vi "Keep time between injections.vi"(6 "Boolean in":bool, 9 "Current Element":string, 10 "Time Target for last measurement in":dbl, 11 "Item Names":string[](array[string])) -> (2 "Boolean out":bool, 3 "Elapsed Time (s)":dbl)   [LabVIEW 2014]
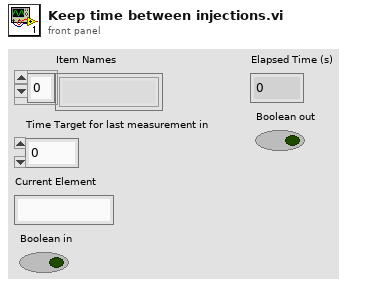
[diagram p1: front panel]
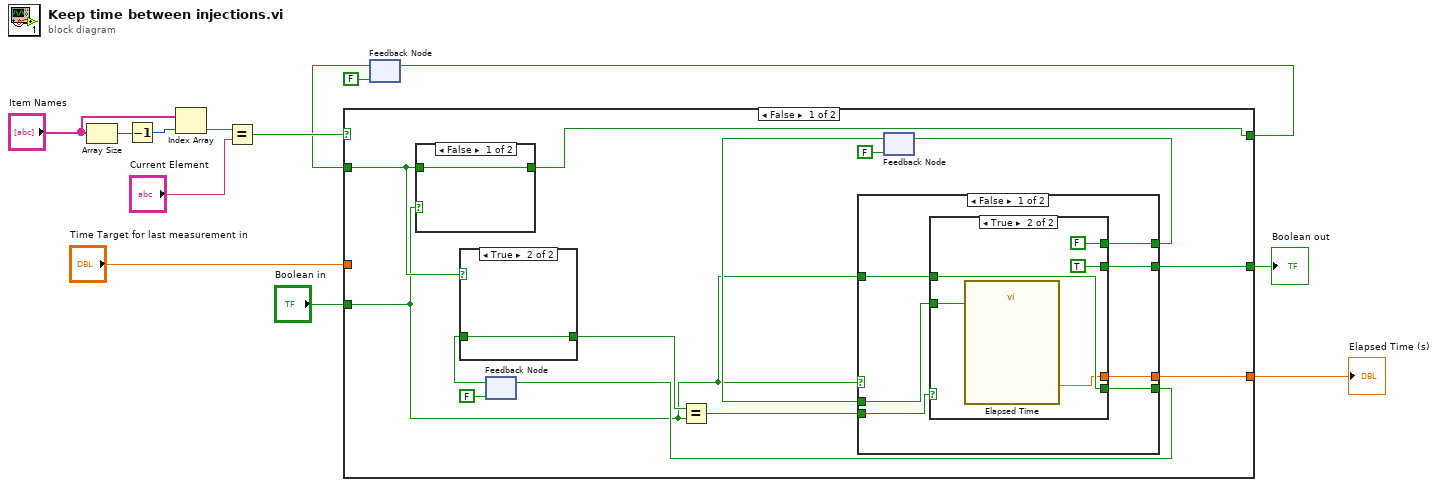
[diagram p0: block diagram]
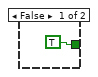
[diagram p2: hidden frame]
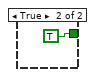
[diagram p3: hidden frame]
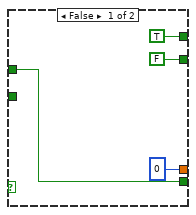
[diagram p4: hidden frame]
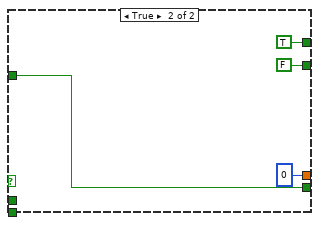
[diagram p5: hidden frame]
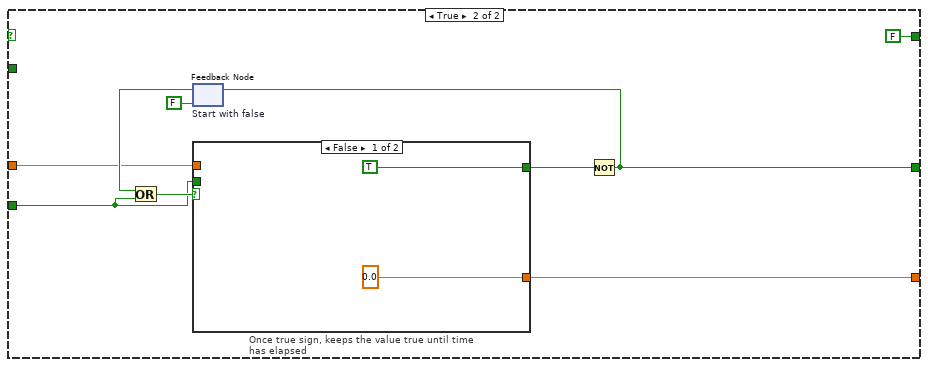
[diagram p6: hidden frame]
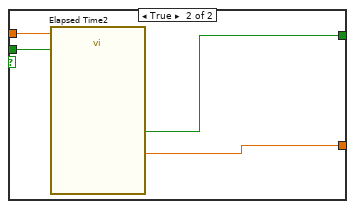
[diagram p7: hidden frame]
diagram:
  n1 = Array Size(array="Item Names") -> (size(s)=w9:i32)
  n2 = Decrement(x=w9) -> (x-1=w10:i32)
  n3 = Index Array(array="Item Names", index=w10) -> (element=w13:string)
  n4 = Equal?(x=w13, y="Current Element") -> (x = y?=w12:bool)
  n5 = feedback #1(FALSE) -> (w6:bool)
  n6 = case shown="False" w12 {
    tunnel: [w25 w56] -> w3
    tunnel: "Boolean in" -> [w14 w54]
    tunnel: "Time Target for last measurement in" -> [_ w51]
    tunnel: w6 -> [w21 _]
    tunnel: [w20 FALSE] -> w7
    tunnel: [w19 w52] -> w8
    frame False {
      n7 = case shown="False" w14 {
        tunnel: w21 -> [w29 _]
        tunnel: [w29 TRUE] -> w20
        frame False {
        }
        frame True {
        }
      }
      n8 = feedback #2(FALSE ("Injection 2")) -> (w22:bool)
      n9 = case shown="True" w21 {
        tunnel: w22 -> [_ w28]
        tunnel: [TRUE w28] -> w18
        frame False {
        }
        frame True {
        }
      }
      n10 = Equal?(x=w18, y=w14) -> (x = y?=w26:bool)
      n11 = feedback #3(FALSE ("Injection 2")) -> (w17:bool)
      n12 = case shown="False" w14 {
        tunnel: w26 -> [w33 _]
        tunnel: [w35 w49] -> w24
        tunnel: w14 -> [w37 w49]
        tunnel: [w36 FALSE] -> w25
        tunnel: [w34 0] -> w19
        tunnel: w17 -> [w31 _]
        tunnel: [w32 TRUE] -> w16
        frame False {
          n13 = case shown="True" w33 {
            tunnel: [w41 w46] -> w35
            tunnel: w37 -> [w41 w46]
            tunnel: [FALSE TRUE] -> w36
            tunnel: [0 w42] -> w34
            tunnel: [TRUE FALSE] -> w32
            tunnel: w31 -> [_ w43]
            frame False {
            }
            frame True {
              n14 = call "Elapsed Time"("Reset"=w43) -> ("Elapsed Time (s)"=w42:dbl)  [unwired: 11 in, 7 out]
            }
          }
        }
        frame True {
        }
      }
      n15 = feedback-in #2(w24) -> ()
      n16 = feedback-in #3(w16) -> ()
    }
    frame True {
      n17 = feedback #4 "Start with false"(FALSE) -> (w55:bool)
      n18 = Or(x=w55, y=w54) -> (x .or. y?=w58:bool)
      n19 = case "Once true sign, keeps the value true until time has elapsed" shown="False" w58 {
        tunnel: w51 -> [_ w65]
        tunnel: [0.0 ("Elapsed Time (s)") w64] -> w52
        tunnel: [TRUE ("Time has Elapsed") w63] -> w59
        tunnel: w54 -> [_ w62]
        frame False {
        }
        frame True {
          n20 = call "Elapsed Time2"("Time Target (s)"=w65, "Reset"=w62) -> ("Elapsed Time (s)"=w64:dbl, "Time has Elapsed"=w63:bool)  [unwired: 10 in, 6 out]
        }
      }
      n21 = Not(x=w59) -> (.not. x?=w56:bool)
      n22 = feedback-in #4(w56) -> ()
    }
  }
  "Elapsed Time (s)" <- w8
  "Boolean out" <- w3
  n23 = feedback-in #1(w7) -> ()
